vi "TCP.IP_Python.vi"(8 "error in (no error)":errorcluster, 10 "loop 1":i32, 11 "Refnum in":refnum<k35>) -> (0 "error out":errorcluster, 2 "Array":dbl[](array[numeric]), 3 "Refnum out":refnum<k35>)   [LabVIEW 2021]
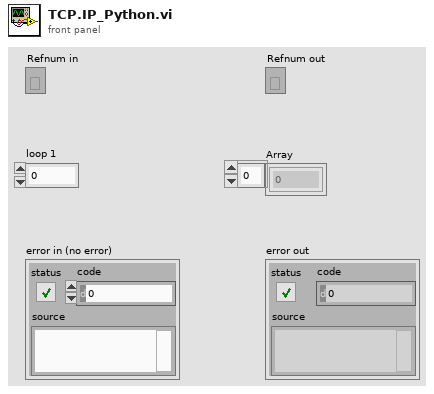
[diagram p1: front panel]
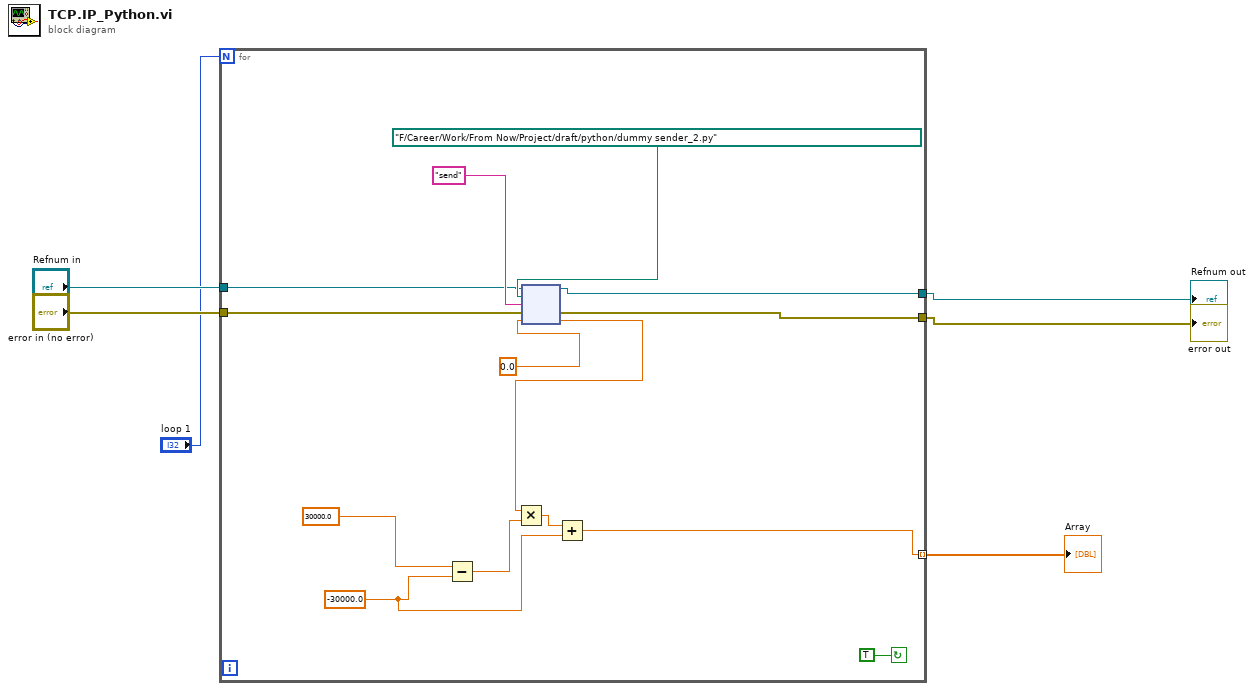
[diagram p0: block diagram]
diagram:
  n1 = for {
    N: "loop 1" -> [_]
    tunnel: [w8] -> w2 mode=indexing
    tunnel: [w18] -> w5
    tunnel: [w17] -> w6
    tunnel: "Refnum in" -> [w16]
    tunnel: "error in (no error)" -> [w15]
    stop <- TRUE continue-if-true
    w11 = -30000.0 ("y")
    n2 = Subtract(x=30000.0, y=w11) -> (x-y=w14:dbl)
    n3 = node(w16, path "F:/Career/Work/From Now/Project/draft/python/dummy sender_2.py" ("module path"), "send" ("function name"), w15, 0.0) -> (w18:refnum<k35>, w17:errorcluster, w9:dbl)  [unwired: 2 out]
    n4 = Multiply(x=w9, y=w14) -> (x*y=w13:dbl)
    n5 = Add(x=w13, y=w11) -> (x+y=w8:dbl)
  }
  "error out" <- w6
  "Refnum out" <- w5
  "Array" <- w2
